vi "PH_Sound.PC _EmergencyOff.vi"(0 "i ref in":refnum<vi>, 3 "State Emernegncy Off":bool, 5 "error in (no error)":errorcluster) -> (14 "i ref out":refnum<vi>, 19 "error out":errorcluster)   [LabVIEW 2014, in "PH_Sound.lvlib"]
doc: "This VI writes the incoming emergency off state to own attributes and the GUI element."
uses:
  PH_Sound.lvlib
  PH_Basics/PH_Common/PH_Common.lvlib
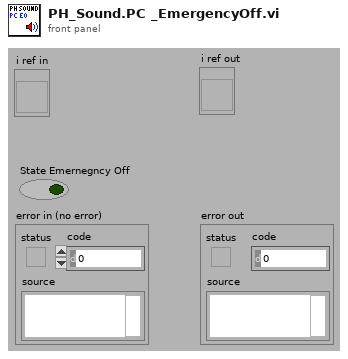
[diagram p1: front panel]
types:
  T1 = typedef "PH_Sound.lvlib/PH_Sound.i attribute.ctl" = cluster{"GUI Refs":cluster{"Exit":refnum<vi>, "Laserfreigabe":refnum<vi>, "PreAmp-Freigabe":refnum<vi>, "Countdown Running":refnum<vi>, "Emergency Off":refnum<vi>, "Device Error":refnum<vi>}, "Testalarm on":bool, "State":cluster{"Laser Class 4":bool, "PreAmp Running":bool, "Countdown Running":bool, "Emergency Off":bool}, "Starting Time":timestamp}
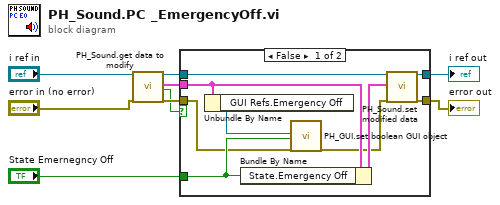
[diagram p0: block diagram]
diagram:
  n1 = call "PH_Sound.get data to modify.vi"("i ref in"="i ref in", "error in (no error)"="error in (no error)") -> ("i ref out"=w3:refnum<vi>, "i attribute"=w2:T1, "timed out"=w1:bool, "error out"=w4:errorcluster)  [unwired: 14 in]
  n2 = case shown="False" w1 {
    tunnel: w4 -> [w11 w19]
    tunnel: w3 -> [w18 w20]
    tunnel: [w17 w20] -> w6
    tunnel: [w16 w19] -> w5
    tunnel: w2 -> [w14 _]
    tunnel: "State Emernegncy Off" -> [w12 _]
    frame False {
      n3 = Unbundle By Name(w14) -> ("GUI Refs.Emergency Off"=w13:refnum<vi>)
      n4 = Bundle By Name(cluster=w14, "State.Emergency Off"=w12) -> (w15:T1)
      n5 = call "PH_GUI.set boolean GUI object.vi"("Boolean Knob GUI Ref"=w13, "Value"=w12, "error in (no error)"=w11) -> ("error out"=w10:errorcluster)  [unwired: 16 in]
      n6 = call "PH_Sound.set modified data.vi"("i ref in"=w18, "i attribute"=w15, "error in (no error)"=w10) -> ("i ref out"=w17:refnum<vi>, "error out"=w16:errorcluster)  [unwired: 15 in]
    }
    frame True {
    }
  }
  "error out" <- w5
  "i ref out" <- w6
